vi "Launch Worker Loop.vi"(8 "error in (no error)":errorcluster, 11 "Asynchronous Application Log in":refnum<class "Asynchronous Application Log.lvclass">) -> (0 "error out":errorcluster, 3 "Asynchronous Application Log out":refnum<class "Asynchronous Application Log.lvclass">)   [LabVIEW 2016, in "Stream Log.lvlib" / "Asynchronous Application Log.lvclass"]
doc: "--\nCopyright © 2017 Composed SystemsI All rights reserved.\n\nAuthor: Jon McBee <jon.mcbee@composed.io>\n\nThis library is provided \"AS IS\" ,WITHOUT WARRANTIES OR\nCONDITIONS OF ANY KIND, either express or implied.\n\nComposed Systems -- composed.io\n\nStream 0.0.1.1\nJon McBee - Composed Systems\nCopyright (c) 2017, Composed Systems"
uses:
  <userlib>/Composed Systems/Stream/Log/Asynchronous Application Log/Asynchronous Application Log.lvclass
  <userlib>/Composed Systems/Stream/Log/Asynchronous Application Log/Message.ctl
  <userlib>/Composed Systems/Stream/Log/Asynchronous Application Log/Entry Type.ctl
  <userlib>/Composed Systems/Stream/Log/Log Sink/Log Sink.lvclass
  <userlib>/Composed Systems/Stream/Log/Asynchronous Application Log/Asynchronous Application Log.lvclass/Asynchronous Application Log.ctl
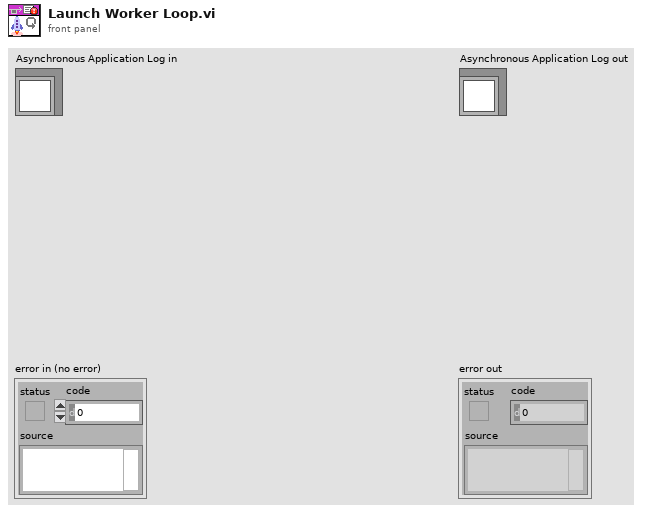
[diagram p1: front panel]
types:
  T1 = typedef "Stream Log.lvlib/Asynchronous Application Log.lvclass/Message.ctl" = cluster{"Entry Type":T2, "String":string, "Sinks":refnum<data-value>[], "Parallel Sinks?":bool}
  T2 = typedef "Stream Log.lvlib/Asynchronous Application Log.lvclass/Entry Type.ctl" = enum16{"Kill Worker", "Log Entry"}
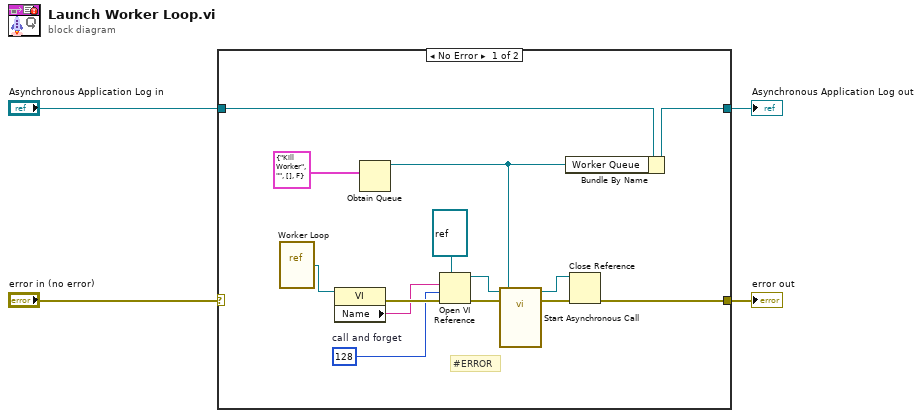
[diagram p0: block diagram]
diagram:
  n1 = case shown="No Error" "error in (no error)" {
    selector: "error in (no error)" -> [_ w20]
    tunnel: [w9 w20] -> w3
    tunnel: [w6 w19] -> w1
    tunnel: "Asynchronous Application Log in" -> [w7 w19]
    frame No Error {
      w15 = 128  # call and forget
      # "#ERROR"
      n2 = vi-ref <userlib>:"Worker Loop.vi"() -> (w18:refnum<vi>)
      n3 = property class="VI"(reference=w18) -> (error out=w17:errorcluster, "Name"=w14:string)  [unwired: 1 in, 1 out]
      n4 = Obtain Queue(element data type=T1 {"Entry Type"=enum."Kill Worker", "String"="", "Sinks"=[], "Parallel Sinks?"=FALSE} ("Message")) -> (queue out=w5:refnum<queue>)  [unwired: 4 in, 2 out]
      n5 = Open VI Reference(type specifier VI Refnum (for type only)=refnum<vi> refnum, vi path=w14, options=w15, error in (no error)=w17) -> (vi reference=w12:refnum<vi>, error out=w13:errorcluster)  [unwired: 2 in]
      n6 = call-by-ref "Start Asynchronous Call"(reference=w12, error in=w13, "Worker Queue"=w5) -> (reference out=w10:refnum<vi>, error out=w11:errorcluster)  [unwired: 11 in]
      n7 = Bundle By Name(cluster=w7, "Worker Queue"=w5) -> (w6:refnum<class "Asynchronous Application Log.lvclass">)
      n8 = Close Reference(reference=w10, error in (no error)=w11) -> (error out=w9:errorcluster)
    }
    frame Error {
    }
  }
  "error out" <- w3
  "Asynchronous Application Log out" <- w1
